vi "get column BLOB.vi"(8 "error in":errorcluster, 9 "column types":i32[](array[ring]) items=["INTEGER"=1, "FLOAT"=2, "STRING"=3, "BLOB"=4, "NULL"=5], 10 "column index":i32, 11 "ppStmt":i64) -> (0 "error out":errorcluster, 1 "column types out":i32[](array[ring]) items=["INTEGER"=1, "FLOAT"=2, "STRING"=3, "BLOB"=4, "NULL"=5], 3 "BLOB":string)   [LabVIEW 2014, in "SQLite3LV.lvlib" / "cursor.lvclass"]
uses:
  cursor.lvclass
  msvcrt.dll
  sqlite3_64.dll
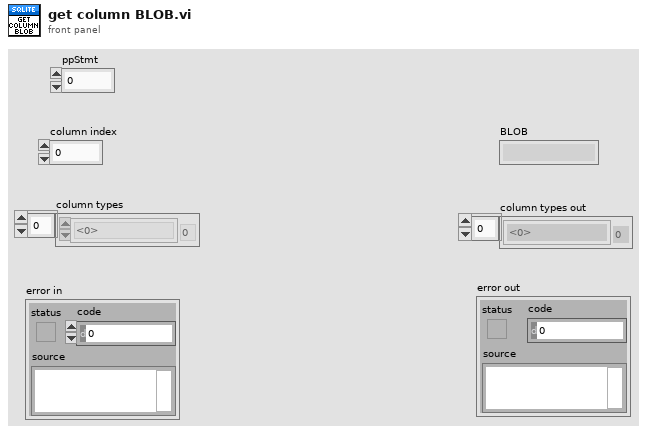
[diagram p1: front panel]
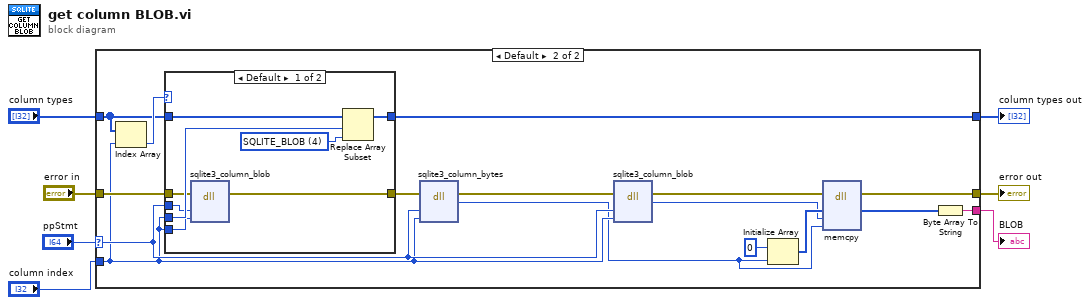
[diagram p0: block diagram]
diagram:
  n1 = case shown="Default" "ppStmt" {
    selector: "ppStmt" -> [_ w19]
    tunnel: [w9 w15] -> w2
    tunnel: "error in" -> [w9 w24]
    tunnel: "column types" -> [w8 w23]
    tunnel: "column index" -> [_ w18]
    tunnel: [_ w11] -> w1
    tunnel: [w8 w21] -> w3
    frame 0 {
    }
    frame Default {
      n2 = Index Array(array=w23, index=w18) -> (element=w25:i32)
      n3 = case shown="Default" w25 {
        tunnel: w24 -> [w29 w35]
        tunnel: [w28 w35] -> w22
        tunnel: w19 -> [w27 _]
        tunnel: w18 -> [w26 _]
        tunnel: w23 -> [w33 w34]
        tunnel: w18 -> [w32 _]
        tunnel: [w30 w34] -> w21
        frame Default {
          w31 = 4 items=["SQLITE_INTEGER"=1, "SQLITE_FLOAT"=2, "SQLITE_TEXT"=3, "SQLITE_BLOB"=4, "SQLITE_NULL"=5] ("new element/subarray")
          n4 = dll-call lib="C:/Users/BobUser/Desktop/LVTables/sqlite3**.*" fn="sqlite3_column_blob"(error in=w29, "pStmt"=w27, "iCol"=w26) -> (error out=w28:errorcluster)  [unwired: 5 in, 1 out]
          n5 = Replace Array Subset(array=w33, new element=w31, index=w32) -> (w30:i32[])
        }
        frame 4 {
        }
      }
      n6 = dll-call lib="C:/Users/BobUser/Desktop/LVTables/sqlite3**.*" fn="sqlite3_column_bytes"(error in=w22, "pStmt"=w19, "iCol"=w18) -> (error out=w20:errorcluster, "num bytes"=w10:i32)  [unwired: 4 in, 1 out]
      n7 = dll-call lib="C:/Users/BobUser/Desktop/LVTables/sqlite3**.*" fn="sqlite3_column_blob"(error in=w20, "pStmt"=w19, "iCol"=w18) -> (error out=w16:errorcluster, "pBytes"=w12:i64)  [unwired: 4 in, 1 out]
      n8 = Initialize Array(u8 0, w10) -> (w13:u8[])
      n9 = dll-call lib="msvcrt.dll" fn="memcpy"(error in=w16, "dest"=w13, "src"=w12, "count"=w10) -> (error out=w15:errorcluster, "dest"=w14:u8[])  [unwired: 5 in, 1 out]
      n10 = Byte Array To String(unsigned byte array=w14) -> (string=w11:string)
    }
  }
  "column types out" <- w3
  "error out" <- w2
  "BLOB" <- w1
